vi "Run.vi"(8 "error in (no error)":errorcluster, 11 "Terminal Message in":refnum<class "Terminal Message.lvclass">) -> (0 "error out":errorcluster, 3 "Terminal Message out":refnum<class "Terminal Message.lvclass">)   [LabVIEW 2016, in "CLD Exam - ATM.lvlib" / "Terminal Message.lvclass"]
uses:
  Terminal Message.lvclass
  D:/Repos/Stream/software/Mediator/Classes/Mediated Actor/Mediated Actor.lvclass
  Mediator/Classes/Message Interface/Message Interface.lvclass
  Terminal Message.lvclass/Terminal Message.ctl
  Log/Application Log/Log Level.ctl
  Mediator/Classes/Message String/Message String.lvclass
  D:/Repos/Stream/software/Mediator/Classes/Message Interface/Message Interface.lvclass
  Mediator/Classes/Message Transport Queue/Message Transport Queue.lvclass
  D:/Repos/Stream/software/Mediator/Classes/Message Transport Interface/Message Transport Interface.lvclass
  Mediator/Classes/Mediated Actor/Mediated Actor.lvclass
  Log/Application Log/Application Log.lvclass
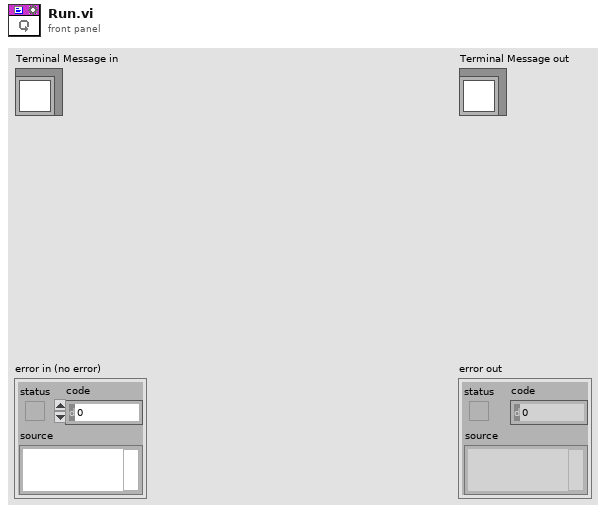
[diagram p1: front panel]
types:
  T1 = cluster{"System Exit":refnum<event-registration>, "Account Action Completed":refnum<event-registration>, "Terminal Timed Out":refnum<event-registration>, "Card Inserted":refnum<event-registration>, "Account Action Requested":refnum<event-registration>, "To Self":refnum<event-registration>}
  T2 = typedef "Stream Log.lvlib/Application Log.lvclass/Log Level.ctl" = enum16{"Imperative", "Major", "Minor", "Debug", "Off"}
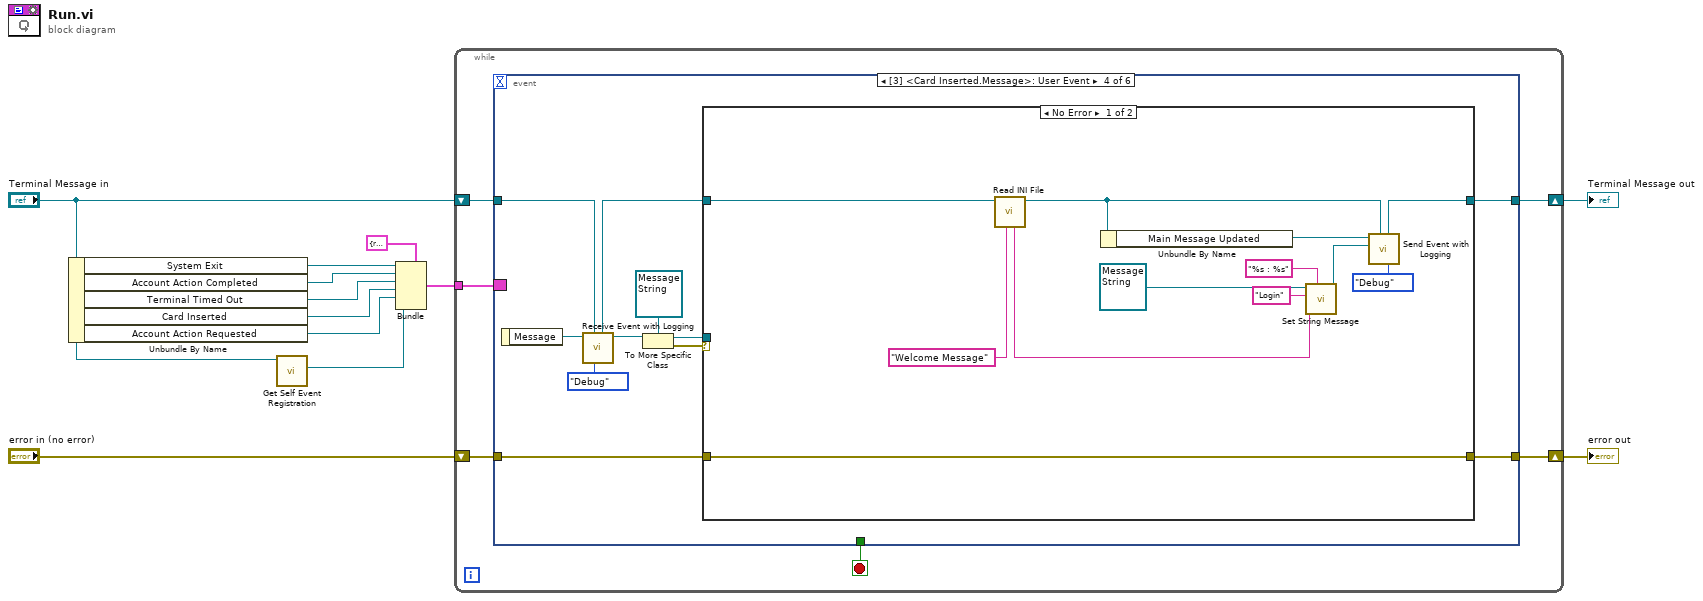
[diagram p0: block diagram]
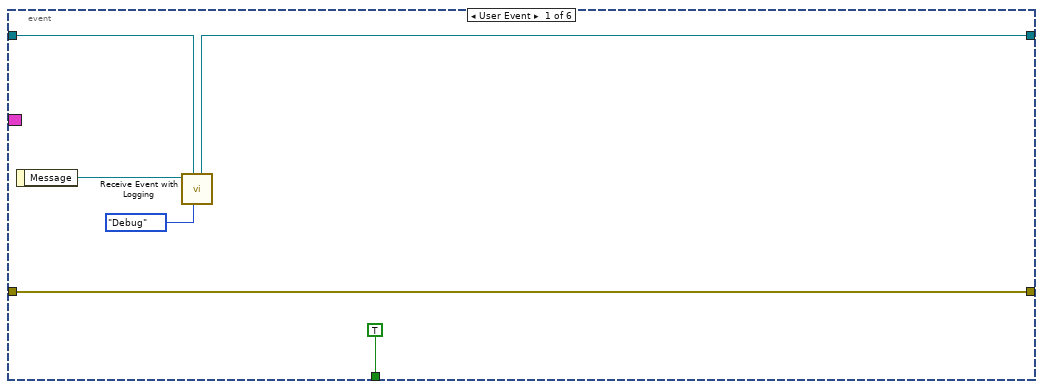
[diagram p2: hidden frame]
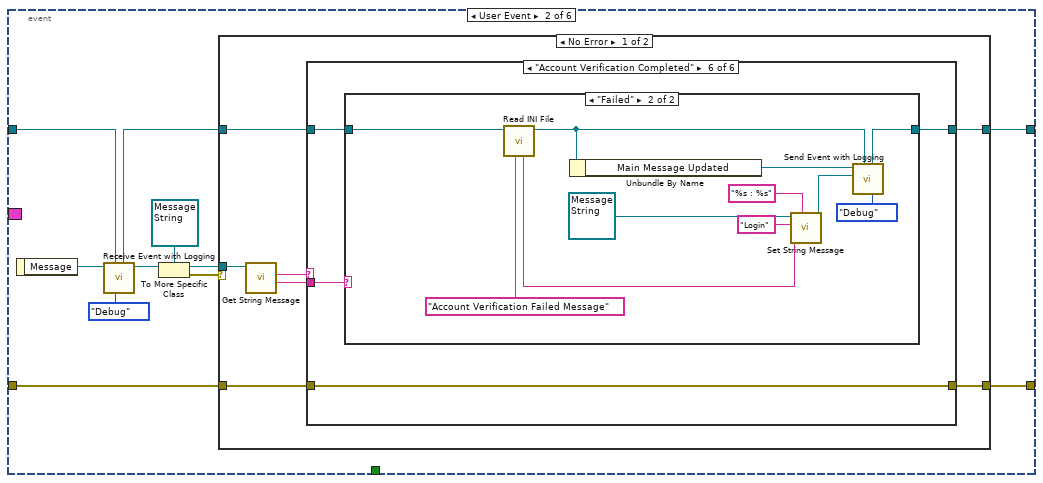
[diagram p3: hidden frame]
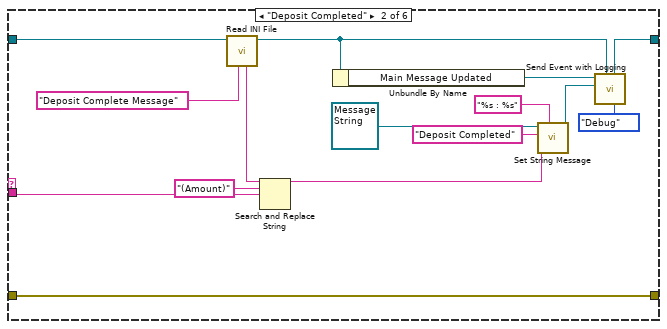
[diagram p5: hidden frame]
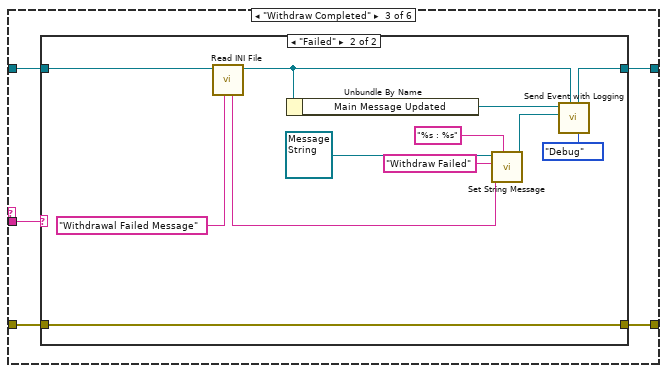
[diagram p6: hidden frame]
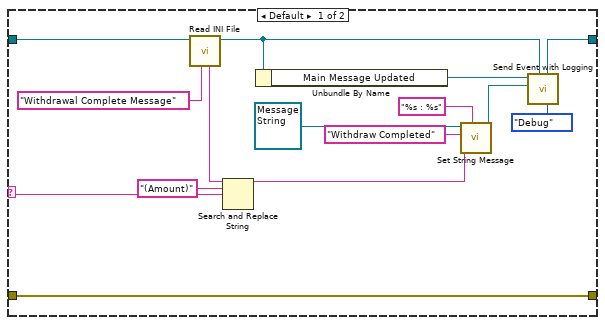
[diagram p7: hidden frame]
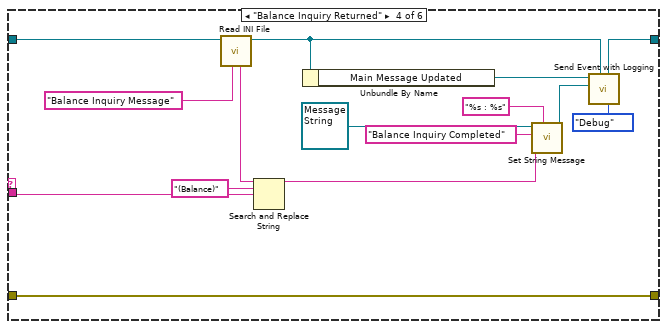
[diagram p8: hidden frame]
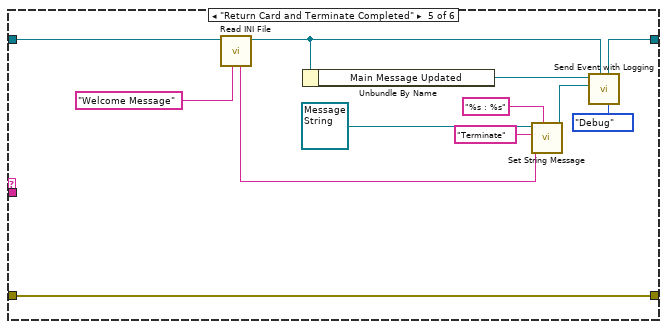
[diagram p9: hidden frame]
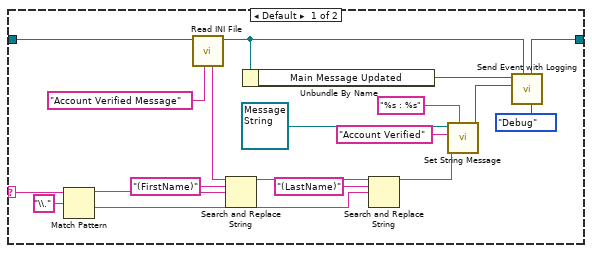
[diagram p10: hidden frame]
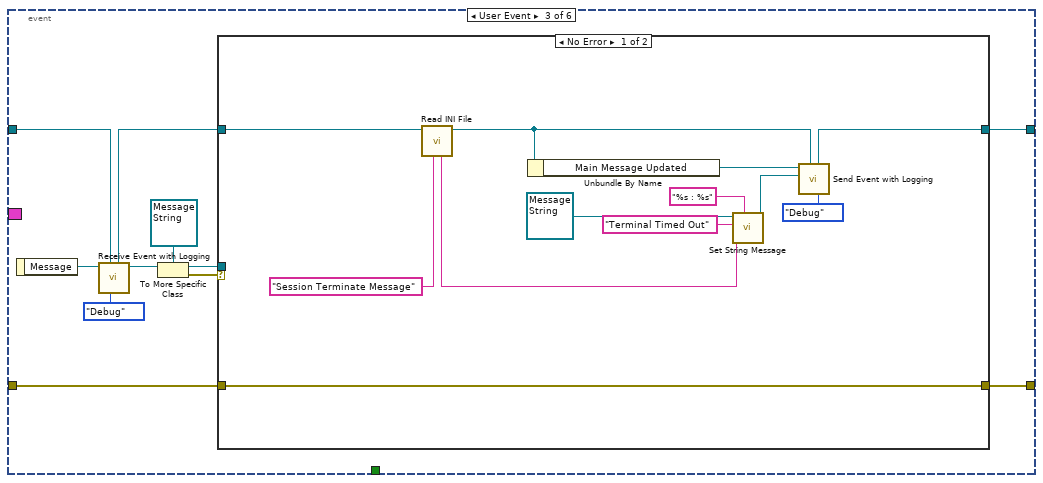
[diagram p12: hidden frame]
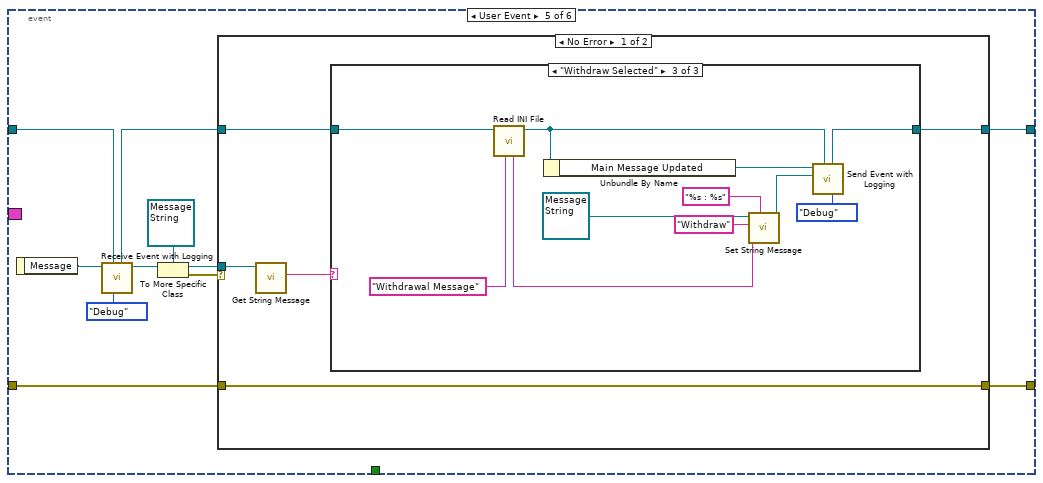
[diagram p15: hidden frame]
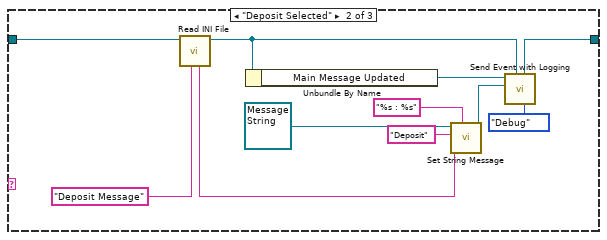
[diagram p17: hidden frame]
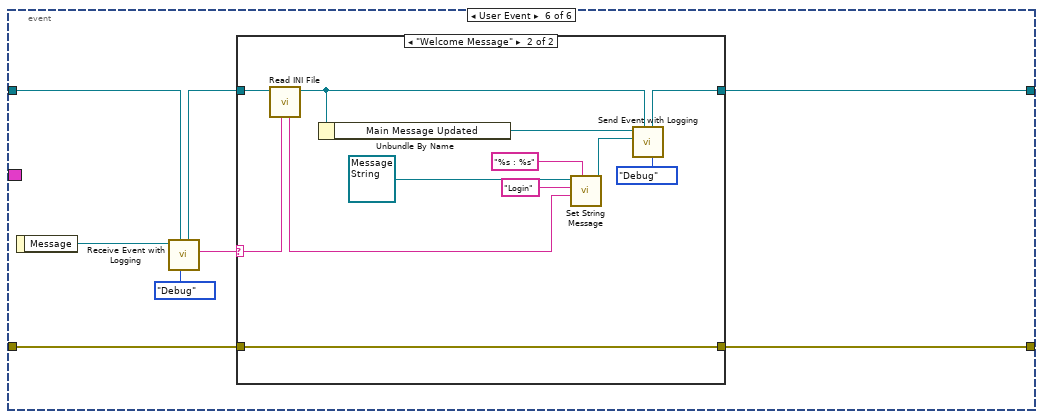
[diagram p19: hidden frame]
diagram:
  n1 = Unbundle By Name("Terminal Message in") -> ("System Exit"=w9:refnum<event-registration>, "Account Action Completed"=w6:refnum<event-registration>, "Terminal Timed Out"=w5:refnum<event-registration>, "Card Inserted"=w4:refnum<event-registration>, "Account Action Requested"=w3:refnum<event-registration>)
  n2 = call "Get Self Event Registration.vi"("Mediated Actor in"="Terminal Message in") -> ("Event Registration Refnum"=w2:refnum<event-registration>)  [unwired: 9 in, 1 out]
  n3 = Bundle(cluster=T1 {"System Exit"=refnum, "Account Action Completed"=refnum, "Terminal Timed Out"=refnum, "Card Inserted"=refnum, "Account Action Requested"=refnum, "To Self"=refnum} ("output cluster"), "System Exit"=w9, "Account Action Completed"=w6, "Terminal Timed Out"=w5, "Card Inserted"=w4, "Account Action Requested"=w3, "To Self"=w2) -> (w7:T1)
  n4 = while {
    shift-right: [w17] -> w12
    shift-left: "Terminal Message in" -> [w18]
    shift-right: [w15] -> w10
    shift-left: "error in (no error)" -> [w16]
    tunnel: w7 -> [w14]
    stop <- w13 stop-if-true
    n5 = event shown="[3] <Card Inserted.Message>: User Event" {
      selector: w14 -> [_ _ _ _ _ _]
      dyn-events: _ -> [_ _ _ _ _ _]
      timeout: _ -> [_ _ _ _ _ _]
      tunnel: w18 -> [w20 w26 w156 w181 w206 w248]
      tunnel: [w19 w32 w162 w187 w212 w253] -> w17
      tunnel: w16 -> [w24 w31 w161 w186 w211 w252]
      tunnel: [w24 w30 w160 w185 w210 w251] -> w15
      tunnel: [TRUE _ _ _ _ _] -> w13
      event User Event {
        n6 = event-data() -> ("Message"=w21:refnum<class "Message Interface.lvclass">)  [unwired: 1 in]
        n7 = call "Receive Event with Logging.vi"("Global Log Level"=Log_Level."Debug", "Mediated Actor in"=w20, "Message"=w21) -> ("Mediated Actor out"=w19:refnum<class "Terminal Message.lvclass">)  [unwired: 5 in, 3 out]
      }
      event User Event {
        n8 = event-data() -> ("Message"=w28:refnum<class "Message Interface.lvclass">)  [unwired: 1 in]
        n9 = call "Receive Event with Logging.vi"("Global Log Level"=Log_Level."Debug", "Mediated Actor in"=w26, "Message"=w28) -> ("Message out"=w27:refnum<class "Message Interface.lvclass">, "Mediated Actor out"=w25:refnum<class "Terminal Message.lvclass">)  [unwired: 5 in, 2 out]
        n10 = To More Specific Class(target class=refnum<class "Message String.lvclass"> refnum ("Message String in"), reference=w27) -> (specific class reference=w34:refnum<class "Message String.lvclass">, error out=w33:errorcluster)  [unwired: 1 in]
        n11 = case shown="No Error" w33 {
          tunnel: w34 -> [w42 _]
          tunnel: [w36 w154] -> w32
          tunnel: w25 -> [w41 w154]
          tunnel: [w39 w153] -> w30
          tunnel: w31 -> [w40 w153]
          frame No Error {
            n12 = call "Get String Message.vi"("Message String in"=w42) -> ("Value"=w37:string, "Name"=w38:string)  [unwired: 7 in, 2 out]
            n13 = case shown="\"Account Verification Completed\"" w38 {
              tunnel: [w44 w45 w63 w92 w108 w120] -> w36
              tunnel: w41 -> [w44 w52 w64 w99 w114 w121]
              tunnel: [w43 w59 w61 w106 w118 w122] -> w39
              tunnel: w40 -> [w43 w59 w62 w106 w118 w122]
              tunnel: w37 -> [_ w51 w60 w98 _ w119]
              frame Default {
              }
              frame "Deposit Completed" {
                n14 = call "Read INI File.vi"("Key"="Deposit Complete Message", "Terminal Message in"=w52) -> ("Terminal Message out"=w46:refnum<class "Terminal Message.lvclass">, "Message"=w55:string)  [unwired: 7 in, 1 out]
                n15 = Search and Replace String(input string=w55, search string="(Amount)", replace string=w51) -> (result string=w54:string)  [unwired: 5 in, 3 out]
                n16 = Unbundle By Name(w46) -> ("Main Message Updated"=w48:refnum<class "Message Transport Queue.lvclass">)
                n17 = call "Set String Message.vi"("Format"="%s : %s", "Value"=w54, "Name"="Deposit Completed", "Message String in"=refnum<class "Message String.lvclass"> refnum) -> ("Message String out"=w47:refnum<class "Message String.lvclass">)  [unwired: 6 in, 1 out]
                n18 = call "Send Event with Logging.vi"("Global Log Level"=Log_Level."Debug", "Mediated Actor in"=w46, "Message"=w47, "Message Transport Interface in"=w48) -> ("Mediated Actor out"=w45:refnum<class "Terminal Message.lvclass">)  [unwired: 6 in, 1 out]
              }
              frame "Withdraw Completed" {
                n19 = case shown="\"Failed\"" w60 {
                  selector: w60 -> [w71 _]
                  tunnel: [w65 w80] -> w63
                  tunnel: w64 -> [w75 w90]
                  tunnel: [w79 w91] -> w61
                  tunnel: w62 -> [w79 w91]
                  frame Default {
                    n20 = call "Read INI File.vi"("Key"="Withdrawal Complete Message", "Terminal Message in"=w75) -> ("Terminal Message out"=w66:refnum<class "Terminal Message.lvclass">, "Message"=w74:string)  [unwired: 7 in, 1 out]
                    n21 = Search and Replace String(input string=w74, search string="(Amount)", replace string=w71) -> (result string=w73:string)  [unwired: 5 in, 3 out]
                    n22 = Unbundle By Name(w66) -> ("Main Message Updated"=w68:refnum<class "Message Transport Queue.lvclass">)
                    n23 = call "Set String Message.vi"("Format"="%s : %s", "Value"=w73, "Name"="Withdraw Completed", "Message String in"=refnum<class "Message String.lvclass"> refnum) -> ("Message String out"=w67:refnum<class "Message String.lvclass">)  [unwired: 6 in, 1 out]
                    n24 = call "Send Event with Logging.vi"("Global Log Level"=Log_Level."Debug", "Mediated Actor in"=w66, "Message"=w67, "Message Transport Interface in"=w68) -> ("Mediated Actor out"=w65:refnum<class "Terminal Message.lvclass">)  [unwired: 6 in, 1 out]
                  }
                  frame "Failed" {
                    n25 = call "Read INI File.vi"("Key"="Withdrawal Failed Message", "Terminal Message in"=w90) -> ("Terminal Message out"=w81:refnum<class "Terminal Message.lvclass">, "Message"=w87:string)  [unwired: 7 in, 1 out]
                    n26 = Unbundle By Name(w81) -> ("Main Message Updated"=w83:refnum<class "Message Transport Queue.lvclass">)
                    n27 = call "Set String Message.vi"("Format"="%s : %s", "Value"=w87, "Name"="Withdraw Failed", "Message String in"=refnum<class "Message String.lvclass"> refnum) -> ("Message String out"=w82:refnum<class "Message String.lvclass">)  [unwired: 6 in, 1 out]
                    n28 = call "Send Event with Logging.vi"("Global Log Level"=Log_Level."Debug", "Mediated Actor in"=w81, "Message"=w82, "Message Transport Interface in"=w83) -> ("Mediated Actor out"=w80:refnum<class "Terminal Message.lvclass">)  [unwired: 6 in, 1 out]
                  }
                }
              }
              frame "Balance Inquiry Returned" {
                n29 = call "Read INI File.vi"("Key"="Balance Inquiry Message", "Terminal Message in"=w99) -> ("Terminal Message out"=w93:refnum<class "Terminal Message.lvclass">, "Message"=w102:string)  [unwired: 7 in, 1 out]
                n30 = Search and Replace String(input string=w102, search string="(Balance)", replace string=w98) -> (result string=w101:string)  [unwired: 5 in, 3 out]
                n31 = Unbundle By Name(w93) -> ("Main Message Updated"=w95:refnum<class "Message Transport Queue.lvclass">)
                n32 = call "Set String Message.vi"("Format"="%s : %s", "Value"=w101, "Name"="Balance Inquiry Completed", "Message String in"=refnum<class "Message String.lvclass"> refnum) -> ("Message String out"=w94:refnum<class "Message String.lvclass">)  [unwired: 6 in, 1 out]
                n33 = call "Send Event with Logging.vi"("Global Log Level"=Log_Level."Debug", "Mediated Actor in"=w93, "Message"=w94, "Message Transport Interface in"=w95) -> ("Mediated Actor out"=w92:refnum<class "Terminal Message.lvclass">)  [unwired: 6 in, 1 out]
              }
              frame "Return Card and Terminate Completed" {
                n34 = call "Read INI File.vi"("Key"="Welcome Message", "Terminal Message in"=w114) -> ("Terminal Message out"=w109:refnum<class "Terminal Message.lvclass">, "Message"=w107:string)  [unwired: 7 in, 1 out]
                n35 = Unbundle By Name(w109) -> ("Main Message Updated"=w111:refnum<class "Message Transport Queue.lvclass">)
                n36 = call "Set String Message.vi"("Format"="%s : %s", "Value"=w107, "Name"="Terminate", "Message String in"=refnum<class "Message String.lvclass"> refnum) -> ("Message String out"=w110:refnum<class "Message String.lvclass">)  [unwired: 6 in, 1 out]
                n37 = call "Send Event with Logging.vi"("Global Log Level"=Log_Level."Debug", "Mediated Actor in"=w109, "Message"=w110, "Message Transport Interface in"=w111) -> ("Mediated Actor out"=w108:refnum<class "Terminal Message.lvclass">)  [unwired: 6 in, 1 out]
              }
              frame "Account Verification Completed" {
                n38 = case shown="\"Failed\"" w119 {
                  selector: w119 -> [w134 _]
                  tunnel: [w123 w142] -> w120
                  tunnel: w121 -> [w138 w152]
                  frame Default {
                    n39 = Match Pattern(string=w134, regular expression="\\.") -> (before substring=w133:string, after substring=w129:string)  [unwired: 1 in, 2 out]
                    n40 = call "Read INI File.vi"("Key"="Account Verified Message", "Terminal Message in"=w138) -> ("Terminal Message out"=w124:refnum<class "Terminal Message.lvclass">, "Message"=w137:string)  [unwired: 7 in, 1 out]
                    n41 = Search and Replace String(input string=w137, search string="(FirstName)", replace string=w133) -> (result string=w131:string)  [unwired: 5 in, 3 out]
                    n42 = Unbundle By Name(w124) -> ("Main Message Updated"=w126:refnum<class "Message Transport Queue.lvclass">)
                    n43 = Search and Replace String(input string=w131, search string="(LastName)", replace string=w129) -> (result string=w130:string)  [unwired: 5 in, 3 out]
                    n44 = call "Set String Message.vi"("Format"="%s : %s", "Value"=w130, "Name"="Account Verified", "Message String in"=refnum<class "Message String.lvclass"> refnum) -> ("Message String out"=w125:refnum<class "Message String.lvclass">)  [unwired: 6 in, 1 out]
                    n45 = call "Send Event with Logging.vi"("Global Log Level"=Log_Level."Debug", "Mediated Actor in"=w124, "Message"=w125, "Message Transport Interface in"=w126) -> ("Mediated Actor out"=w123:refnum<class "Terminal Message.lvclass">)  [unwired: 6 in, 1 out]
                  }
                  frame "Failed" {
                    n46 = call "Read INI File.vi"("Key"="Account Verification Failed Message", "Terminal Message in"=w152) -> ("Terminal Message out"=w143:refnum<class "Terminal Message.lvclass">, "Message"=w149:string)  [unwired: 7 in, 1 out]
                    n47 = Unbundle By Name(w143) -> ("Main Message Updated"=w145:refnum<class "Message Transport Queue.lvclass">)
                    n48 = call "Set String Message.vi"("Format"="%s : %s", "Value"=w149, "Name"="Login", "Message String in"=refnum<class "Message String.lvclass"> refnum) -> ("Message String out"=w144:refnum<class "Message String.lvclass">)  [unwired: 6 in, 1 out]
                    n49 = call "Send Event with Logging.vi"("Global Log Level"=Log_Level."Debug", "Mediated Actor in"=w143, "Message"=w144, "Message Transport Interface in"=w145) -> ("Mediated Actor out"=w142:refnum<class "Terminal Message.lvclass">)  [unwired: 6 in, 1 out]
                  }
                }
              }
            }
          }
          frame Error {
          }
        }
      }
      event User Event {
        n50 = event-data() -> ("Message"=w158:refnum<class "Message Interface.lvclass">)  [unwired: 1 in]
        n51 = call "Receive Event with Logging.vi"("Global Log Level"=Log_Level."Debug", "Mediated Actor in"=w156, "Message"=w158) -> ("Message out"=w157:refnum<class "Message Interface.lvclass">, "Mediated Actor out"=w155:refnum<class "Terminal Message.lvclass">)  [unwired: 5 in, 2 out]
        n52 = To More Specific Class(target class=refnum<class "Message String.lvclass"> refnum ("Message String in"), reference=w157) -> (specific class reference=w164:refnum<class "Message String.lvclass">, error out=w163:errorcluster)  [unwired: 1 in]
        n53 = case shown="No Error" w163 {
          tunnel: w164 -> [_ _]
          tunnel: [w166 w179] -> w162
          tunnel: w155 -> [w177 w179]
          tunnel: [w176 w178] -> w160
          tunnel: w161 -> [w176 w178]
          frame No Error {
            n54 = call "Read INI File.vi"("Key"="Session Terminate Message", "Terminal Message in"=w177) -> ("Terminal Message out"=w167:refnum<class "Terminal Message.lvclass">, "Message"=w173:string)  [unwired: 7 in, 1 out]
            n55 = Unbundle By Name(w167) -> ("Main Message Updated"=w169:refnum<class "Message Transport Queue.lvclass">)
            n56 = call "Set String Message.vi"("Format"="%s : %s", "Value"=w173, "Name"="Terminal Timed Out", "Message String in"=refnum<class "Message String.lvclass"> refnum) -> ("Message String out"=w168:refnum<class "Message String.lvclass">)  [unwired: 6 in, 1 out]
            n57 = call "Send Event with Logging.vi"("Global Log Level"=Log_Level."Debug", "Mediated Actor in"=w167, "Message"=w168, "Message Transport Interface in"=w169) -> ("Mediated Actor out"=w166:refnum<class "Terminal Message.lvclass">)  [unwired: 6 in, 1 out]
          }
          frame Error {
          }
        }
      }
      event User Event {
        n58 = event-data() -> ("Message"=w183:refnum<class "Message Interface.lvclass">)  [unwired: 1 in]
        n59 = call "Receive Event with Logging.vi"("Global Log Level"=Log_Level."Debug", "Mediated Actor in"=w181, "Message"=w183) -> ("Message out"=w182:refnum<class "Message Interface.lvclass">, "Mediated Actor out"=w180:refnum<class "Terminal Message.lvclass">)  [unwired: 5 in, 2 out]
        n60 = To More Specific Class(target class=refnum<class "Message String.lvclass"> refnum ("Message String in"), reference=w182) -> (specific class reference=w189:refnum<class "Message String.lvclass">, error out=w188:errorcluster)  [unwired: 1 in]
        n61 = case shown="No Error" w188 {
          tunnel: w189 -> [_ _]
          tunnel: [w191 w204] -> w187
          tunnel: w180 -> [w202 w204]
          tunnel: [w201 w203] -> w185
          tunnel: w186 -> [w201 w203]
          frame No Error {
            n62 = call "Read INI File.vi"("Key"="Welcome Message", "Terminal Message in"=w202) -> ("Terminal Message out"=w192:refnum<class "Terminal Message.lvclass">, "Message"=w198:string)  [unwired: 7 in, 1 out]
            n63 = Unbundle By Name(w192) -> ("Main Message Updated"=w194:refnum<class "Message Transport Queue.lvclass">)
            n64 = call "Set String Message.vi"("Format"="%s : %s", "Value"=w198, "Name"="Login", "Message String in"=refnum<class "Message String.lvclass"> refnum) -> ("Message String out"=w193:refnum<class "Message String.lvclass">)  [unwired: 6 in, 1 out]
            n65 = call "Send Event with Logging.vi"("Global Log Level"=Log_Level."Debug", "Mediated Actor in"=w192, "Message"=w193, "Message Transport Interface in"=w194) -> ("Mediated Actor out"=w191:refnum<class "Terminal Message.lvclass">)  [unwired: 6 in, 1 out]
          }
          frame Error {
          }
        }
      }
      event User Event {
        n66 = event-data() -> ("Message"=w208:refnum<class "Message Interface.lvclass">)  [unwired: 1 in]
        n67 = call "Receive Event with Logging.vi"("Global Log Level"=Log_Level."Debug", "Mediated Actor in"=w206, "Message"=w208) -> ("Message out"=w207:refnum<class "Message Interface.lvclass">, "Mediated Actor out"=w205:refnum<class "Terminal Message.lvclass">)  [unwired: 5 in, 2 out]
        n68 = To More Specific Class(target class=refnum<class "Message String.lvclass"> refnum ("Message String in"), reference=w207) -> (specific class reference=w214:refnum<class "Message String.lvclass">, error out=w213:errorcluster)  [unwired: 1 in]
        n69 = case shown="No Error" w213 {
          tunnel: w214 -> [w217 _]
          tunnel: [w218 w245] -> w212
          tunnel: w205 -> [w220 w245]
          tunnel: [w219 w244] -> w210
          tunnel: w211 -> [w219 w244]
          frame No Error {
            n70 = call "Get String Message.vi"("Message String in"=w217) -> ("Name"=w216:string)  [unwired: 7 in, 3 out]
            n71 = case shown="\"Withdraw Selected\"" w216 {
              tunnel: w220 -> [w221 w227 w238]
              tunnel: [w221 w222 w233] -> w218
              frame Default {
              }
              frame "Deposit Selected" {
                n72 = call "Read INI File.vi"("Key"="Deposit Message", "Terminal Message in"=w227) -> ("Terminal Message out"=w223:refnum<class "Terminal Message.lvclass">, "Message"=w230:string)  [unwired: 7 in, 1 out]
                n73 = Unbundle By Name(w223) -> ("Main Message Updated"=w225:refnum<class "Message Transport Queue.lvclass">)
                n74 = call "Set String Message.vi"("Format"="%s : %s", "Value"=w230, "Name"="Deposit", "Message String in"=refnum<class "Message String.lvclass"> refnum) -> ("Message String out"=w224:refnum<class "Message String.lvclass">)  [unwired: 6 in, 1 out]
                n75 = call "Send Event with Logging.vi"("Global Log Level"=Log_Level."Debug", "Mediated Actor in"=w223, "Message"=w224, "Message Transport Interface in"=w225) -> ("Mediated Actor out"=w222:refnum<class "Terminal Message.lvclass">)  [unwired: 6 in, 1 out]
              }
              frame "Withdraw Selected" {
                n76 = call "Read INI File.vi"("Key"="Withdrawal Message", "Terminal Message in"=w238) -> ("Terminal Message out"=w234:refnum<class "Terminal Message.lvclass">, "Message"=w241:string)  [unwired: 7 in, 1 out]
                n77 = Unbundle By Name(w234) -> ("Main Message Updated"=w236:refnum<class "Message Transport Queue.lvclass">)
                n78 = call "Set String Message.vi"("Format"="%s : %s", "Value"=w241, "Name"="Withdraw", "Message String in"=refnum<class "Message String.lvclass"> refnum) -> ("Message String out"=w235:refnum<class "Message String.lvclass">)  [unwired: 6 in, 1 out]
                n79 = call "Send Event with Logging.vi"("Global Log Level"=Log_Level."Debug", "Mediated Actor in"=w234, "Message"=w235, "Message Transport Interface in"=w236) -> ("Mediated Actor out"=w233:refnum<class "Terminal Message.lvclass">)  [unwired: 6 in, 1 out]
              }
            }
          }
          frame Error {
          }
        }
      }
      event User Event {
        n80 = event-data() -> ("Message"=w250:refnum<class "Message Interface.lvclass">)  [unwired: 1 in]
        n81 = call "Receive Event with Logging.vi"("Global Log Level"=Log_Level."Debug", "Mediated Actor in"=w248, "Message"=w250) -> ("Name"=w249:string, "Mediated Actor out"=w247:refnum<class "Terminal Message.lvclass">)  [unwired: 5 in, 2 out]
        n82 = case shown="\"Welcome Message\"" w249 {
          selector: w249 -> [_ w265]
          tunnel: [w255 w256] -> w253
          tunnel: w247 -> [w255 w266]
          tunnel: [w254 w267] -> w251
          tunnel: w252 -> [w254 w267]
          frame Default {
          }
          frame "Welcome Message" {
            n83 = call "Read INI File.vi"("Key"=w265, "Terminal Message in"=w266) -> ("Terminal Message out"=w257:refnum<class "Terminal Message.lvclass">, "Message"=w262:string)  [unwired: 7 in, 1 out]
            n84 = Unbundle By Name(w257) -> ("Main Message Updated"=w259:refnum<class "Message Transport Queue.lvclass">)
            n85 = call "Set String Message.vi"("Format"="%s : %s", "Value"=w262, "Name"="Login", "Message String in"=refnum<class "Message String.lvclass"> refnum) -> ("Message String out"=w258:refnum<class "Message String.lvclass">)  [unwired: 6 in, 1 out]
            n86 = call "Send Event with Logging.vi"("Global Log Level"=Log_Level."Debug", "Mediated Actor in"=w257, "Message"=w258, "Message Transport Interface in"=w259) -> ("Mediated Actor out"=w256:refnum<class "Terminal Message.lvclass">)  [unwired: 6 in, 1 out]
          }
        }
      }
    }
  }
  "error out" <- w10
  "Terminal Message out" <- w12
